vi "Extract Stability Parameters.vi"(11 "Programmer Step":T1) -> (1 "Ranges":dbl[](array[numeric]), 3 "Setpoints":dbl[](array[numeric]))   [LabVIEW 2012]
uses:
  Data Types/Programmer Step.ctl
  Data Types/Programmer Step References.ctl
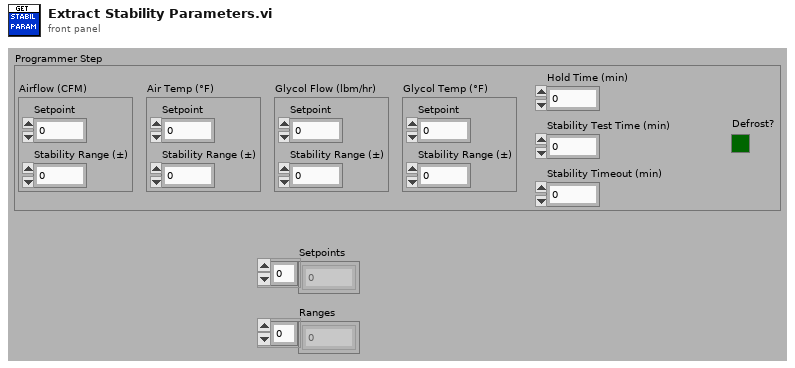
[diagram p1: front panel]
types:
  T1 = typedef "Programmer Step.ctl" = cluster{"Airflow (CFM)":T2, "Air Temp (°F)":T2, "Glycol Flow (lbm/hr)":T2, "Glycol Temp (°F)":T2, "Hold Time (min)":dbl, "Stability Test Time (min)":dbl, "Stability Timeout (min)":dbl, "Defrost?":bool}
  T2 = typedef "Programmer Step References.ctl" = cluster{"Setpoint":dbl, "Stability Range (±)":dbl}
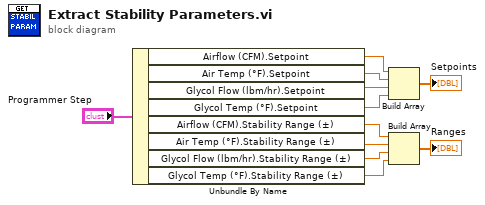
[diagram p0: block diagram]
diagram:
  n1 = Unbundle By Name("Programmer Step") -> ("Airflow (CFM).Setpoint"=w4:dbl, "Air Temp (°F).Setpoint"=w5:dbl, "Glycol Flow (lbm/hr).Setpoint"=w6:dbl, "Glycol Temp (°F).Setpoint"=w7:dbl, "Airflow (CFM).Stability Range (±)"=w8:dbl, "Air Temp (°F).Stability Range (±)"=w9:dbl, "Glycol Flow (lbm/hr).Stability Range (±)"=w10:dbl, "Glycol Temp (°F).Stability Range (±)"=w11:dbl)
  n2 = Build Array(w4, w5, w6, w7) -> (→"Setpoints":dbl[])
  n3 = Build Array(w8, w9, w10, w11) -> (→"Ranges":dbl[])
